vi "Draw Comparison.vi"(5 "Best Fit Parameters":dbl[](array[numeric]), 7 "Best Fit":dbl[][](array[numeric]), 10 "Raw Data":dbl[][](array[numeric])) -> (0 "Horizontal Comparison":cluster{i32[], dbl[]}[](graph), 3 "Vertical Comparison":cluster{i32[], dbl[]}[](graph))   [LabVIEW 2015]
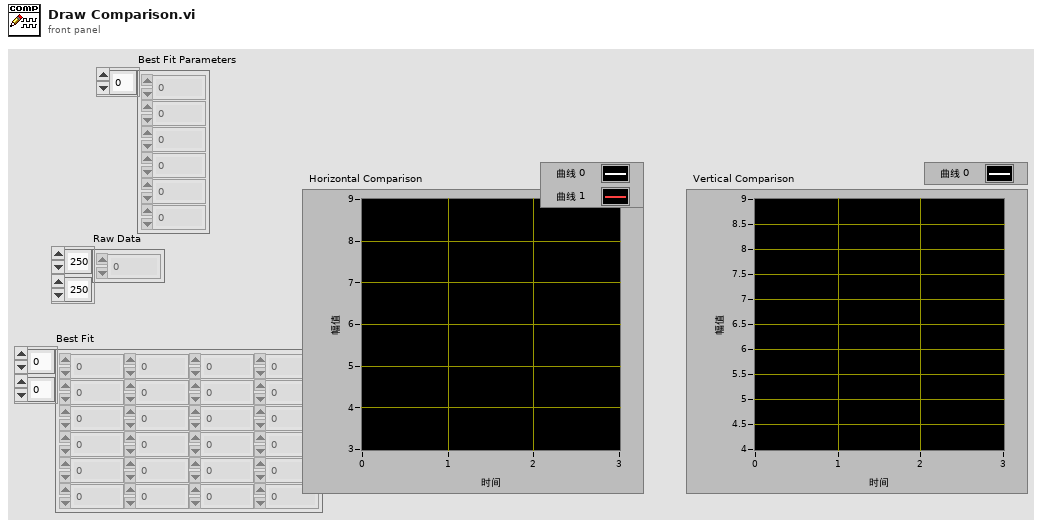
[diagram p1: front panel]
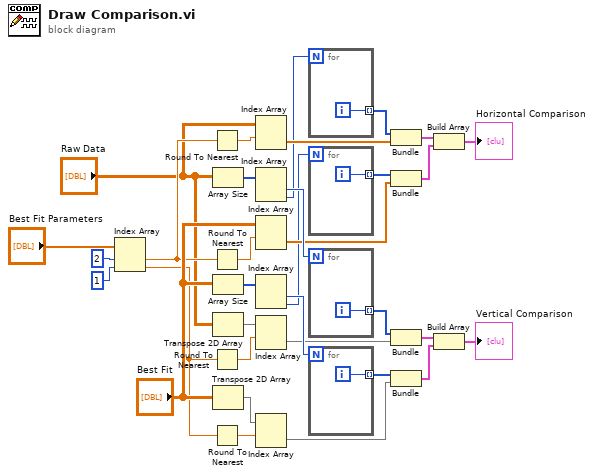
[diagram p0: block diagram]
diagram:
  n1 = Index Array(array="Best Fit Parameters", index #1=2 ("index"), index #2=1 ("index")) -> (element #1=w2:dbl, element #2=w3:dbl)
  n2 = Round To Nearest(number=w2) -> (nearest integer value=w14:dbl)
  n3 = Round To Nearest(number=w2) -> (nearest integer value=w19:dbl)
  n4 = Round To Nearest(number=w3) -> (nearest integer value=w16:dbl)
  n5 = Round To Nearest(number=w3) -> (nearest integer value=w7:dbl)
  n6 = Array Size(array="Raw Data") -> (size(s)=w26:i32[])
  n7 = Array Size(array="Best Fit") -> (size(s)=w24:i32[])
  n8 = Transpose 2D Array(2D array="Raw Data") -> (transposed array=w17:dbl[][])
  n9 = Transpose 2D Array(2D array="Best Fit") -> (transposed array=w22:dbl[][])
  n10 = Index Array(array="Raw Data", index (row)=w14) -> (element=w13:dbl[])  [unwired: 1 in]
  n11 = Index Array(array=w26) -> (element #1=w25:i32, element #2=w8:i32)  [unwired: 2 in]
  n12 = Index Array(array="Best Fit", index (row)=w19) -> (element=w18:dbl[])  [unwired: 1 in]
  n13 = Index Array(array=w24) -> (element #1=w23:i32, element #2=w9:i32)  [unwired: 2 in]
  n14 = Index Array(array=w17, index (row)=w16) -> (element=w15:dbl[])  [unwired: 1 in]
  n15 = Index Array(array=w22, index (row)=w7) -> (element=w21:dbl[])  [unwired: 1 in]
  n16 = for {
    N: w8 -> [_]
    tunnel: [w34] -> w30 mode=indexing
    i -> [w34]
  }
  n17 = for {
    N: w9 -> [_]
    tunnel: [w35] -> w32 mode=indexing
    i -> [w35]
  }
  n18 = for {
    N: w25 -> [_]
    tunnel: [w36] -> w31 mode=indexing
    i -> [w36]
  }
  n19 = for {
    N: w23 -> [_]
    tunnel: [w37] -> w33 mode=indexing
    i -> [w37]
  }
  n20 = Bundle(w30, "Raw Data"=w13) -> (w29:cluster{i32[], "Raw Data":dbl[]})  [unwired: 1 in]
  n21 = Bundle(w32, "Best Fit"=w18) -> (w28:cluster{i32[], "Best Fit":dbl[]})  [unwired: 1 in]
  n22 = Bundle(w31, w15) -> (w27:cluster{i32[], dbl[]})  [unwired: 1 in]
  n23 = Bundle(w33, w21) -> (w12:cluster{i32[], dbl[]})  [unwired: 1 in]
  n24 = Build Array(w29, w28) -> (→"Horizontal Comparison":cluster{i32[], "Best Fit":dbl[]}[])
  n25 = Build Array(w27, w12) -> (→"Vertical Comparison":cluster{i32[], dbl[]}[])
